vi "ble_discover_services.vi"(5 "Last Handle Number (0xFFFF)":u16=65535 format="%04x", 6 "Connection Status":T2={"MAC Address"="", "cnx handle"=0, "cnx flags"=0, "Address Type"=125, "Connection Interval (ms)"=125, "Timeout(ms)"=125, "Latency"=0, "bonding handle"=0} {"Address Type" items=["Public", "Random"]}, 7 "First Handle Number(0x0001)":u16=1 format="%04x", 8 "error in (no error)":errorcluster, 11 "COM Bluegiga in":refnum<visa-resource-name>) -> (0 "error out":errorcluster, 2 "service_info":u8[][](array[numeric]), 3 "COM Bluegiga out":refnum<visa-resource-name>)   [LabVIEW 2013]
uses:
  type_def/connection_status_bundle.ctl
  type_def/address_type.ctl
  type_def/service_type.ctl
panel:
  in  "Service Type (0x2800)":T1=10240 format="%04x" items=["Primary"=10240, "Secundary"=10241]
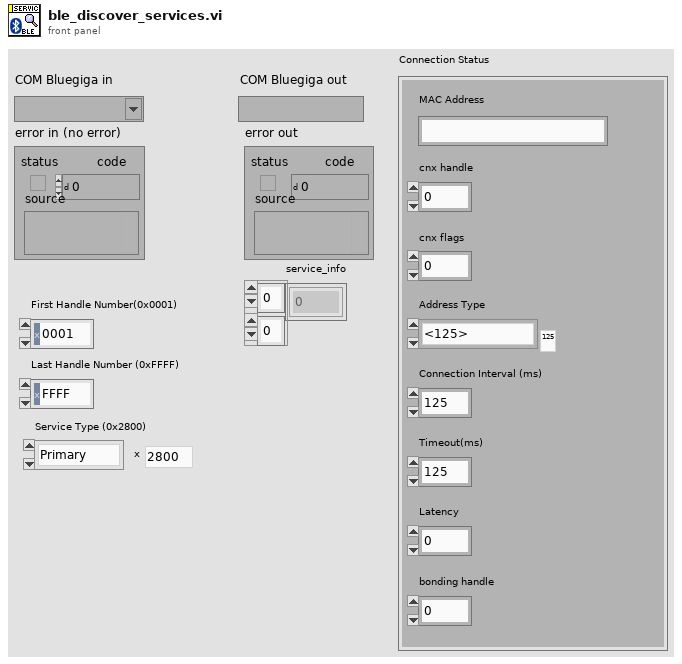
[diagram p1: front panel]
types:
  T1 = typedef "service_type.ctl" = u16
  T2 = typedef "connection_status_bundle.ctl" = cluster{"MAC Address":string, "cnx handle":u8, "cnx flags":u8, "Address Type":T3, "Connection Interval (ms)":u16, "Timeout(ms)":u16, "Latency":u16, "bonding handle":u8}
  T3 = typedef "address_type.ctl" = u8
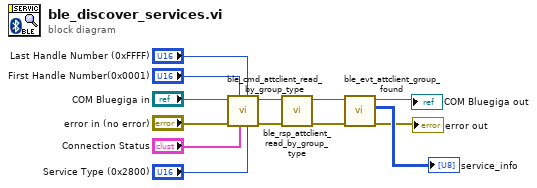
[diagram p0: block diagram]
diagram:
  n1 = call "ble_cmd_attclient_read_by_group_type.vi"("Service Type (0x2800)"="Service Type (0x2800)", "Last Handle Number (0xFFFF)"="Last Handle Number (0xFFFF)", "Connection Status"="Connection Status", "First Handle Number(0x0001)"="First Handle Number(0x0001)", "error in (no error)"="error in (no error)", "COM Bluegiga in"="COM Bluegiga in") -> ("error out"=w10:errorcluster, "COM Bluegiga out"=w12:refnum<visa-resource-name>)  [unwired: 4 in]
  n2 = call "ble_rsp_attclient_read_by_group_type.vi"("error in (no error)"=w10, "COM Bluegiga in"=w12) -> ("error out"=w11:errorcluster, "COM Bluegiga out"=w13:refnum<visa-resource-name>)  [unwired: 6 in, 2 out]
  n3 = call "ble_evt_attclient_group_found.vi"("error in (no error)"=w11, "COM Bluegiga in"=w13) -> ("error out"=→"error out":errorcluster, "service_info"=→"service_info":u8[][], "COM Bluegiga out"=→"COM Bluegiga out":refnum<visa-resource-name>)  [unwired: 7 in]
